vi "CALC_Pix_to_zone_correspondence.vi"(2 "Array of the pixel to color correspondences":u32[][](array[numeric]), 3 "Array of the zone to color correspondences":u32[][](array[numeric])) -> (1 "Array of the pixel to zone correspondences":T1)   [LabVIEW 2018, in "Tracker.lvlib"]
uses:
  Tracker.lvlib
  Controls/CTL_Pixel_to_Zone_array.ctl
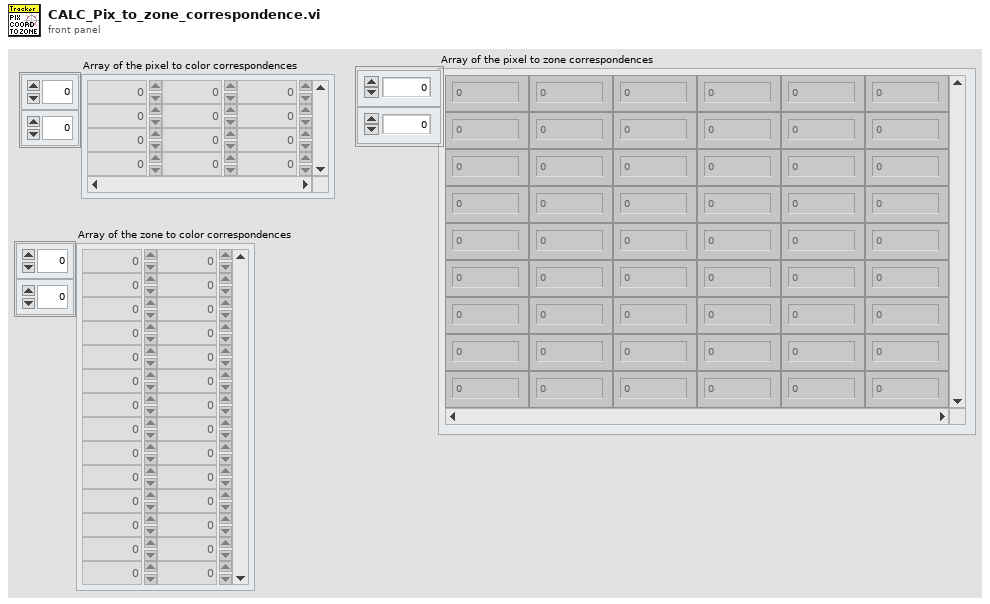
[diagram p1: front panel]
types:
  T1 = typedef "Tracker.lvlib/CTL_Pixel_to_Zone_array.ctl" = i8[][]
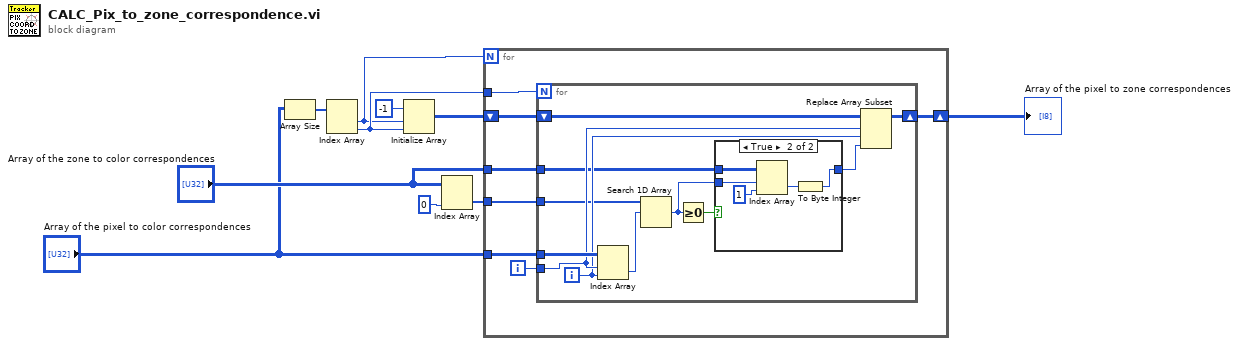
[diagram p0: block diagram]
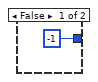
[diagram p2: hidden frame]
diagram:
  n1 = Array Size(array="Array of the pixel to color correspondences") -> (size(s)=w1:i32[])
  n2 = Index Array(array=w1) -> (element #1=w8:i32, element #2=w9:i32)  [unwired: 2 in]
  n3 = Initialize Array(i8 -1, w8, w9) -> (w3:i8[][])
  n4 = Index Array(array="Array of the zone to color correspondences", index (col)=0 ("index (row)")) -> (element=w6:u32[])  [unwired: 1 in]
  n5 = for {
    N: w8 -> [_]
    tunnel: "Array of the pixel to color correspondences" -> [w17]
    shift-right: [w15] -> w4
    shift-left: w3 -> [w16]
    tunnel: w6 -> [w13]
    tunnel: "Array of the zone to color correspondences" -> [w12]
    tunnel: w9 -> [w11]
    i -> [w14]
    n6 = for {
      N: w11 -> [_]
      tunnel: w17 -> [w27]
      shift-right: [w20] -> w15
      shift-left: w16 -> [w28]
      tunnel: w14 -> [w26]
      tunnel: w13 -> [w24]
      tunnel: w12 -> [w22]
      i -> [w25]
      n7 = Index Array(array=w27, index (row)=w26, index (col)=w25) -> (element=w23:u32)
      n8 = Search 1D Array(1D array=w24, element=w23) -> (index of element=w18:i32)  [unwired: 1 in]
      n9 = Greater Or Equal To 0?(x=w18) -> (x >= 0?=w19:bool)
      n10 = case shown="True" w19 {
        tunnel: w22 -> [_ w34]
        tunnel: w18 -> [_ w33]
        tunnel: [i8 -1 ("Color for central segment") w30] -> w21
        frame False {
        }
        frame True {
          n11 = Index Array(array=w34, index (row)=w33, index (col)=1 ("disabled index (col)")) -> (element=w31:u32)
          n12 = To Byte Integer(number=w31) -> (8bit integer=w30:i8)
        }
      }
      n13 = Replace Array Subset(array=w28, new element=w21, index (row)=w26, index (col)=w25) -> (w20:i8[][])
    }
  }
  "Array of the pixel to zone correspondences" <- w4
